vi "Day 11-1.vi"() -> ()   [LabVIEW 2020]
uses:
  <vilib>/regexp/Match Regular Expression.xnode
panel:
  out "Answer":i64
  out "Array":i32[][](array[numeric])
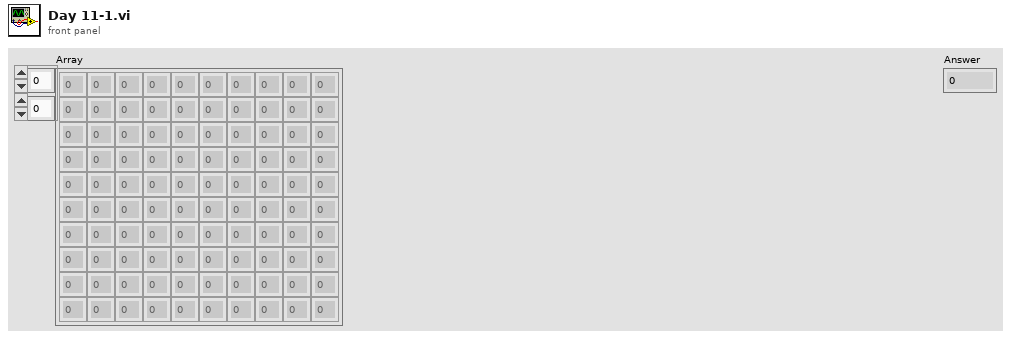
[diagram p1: front panel]
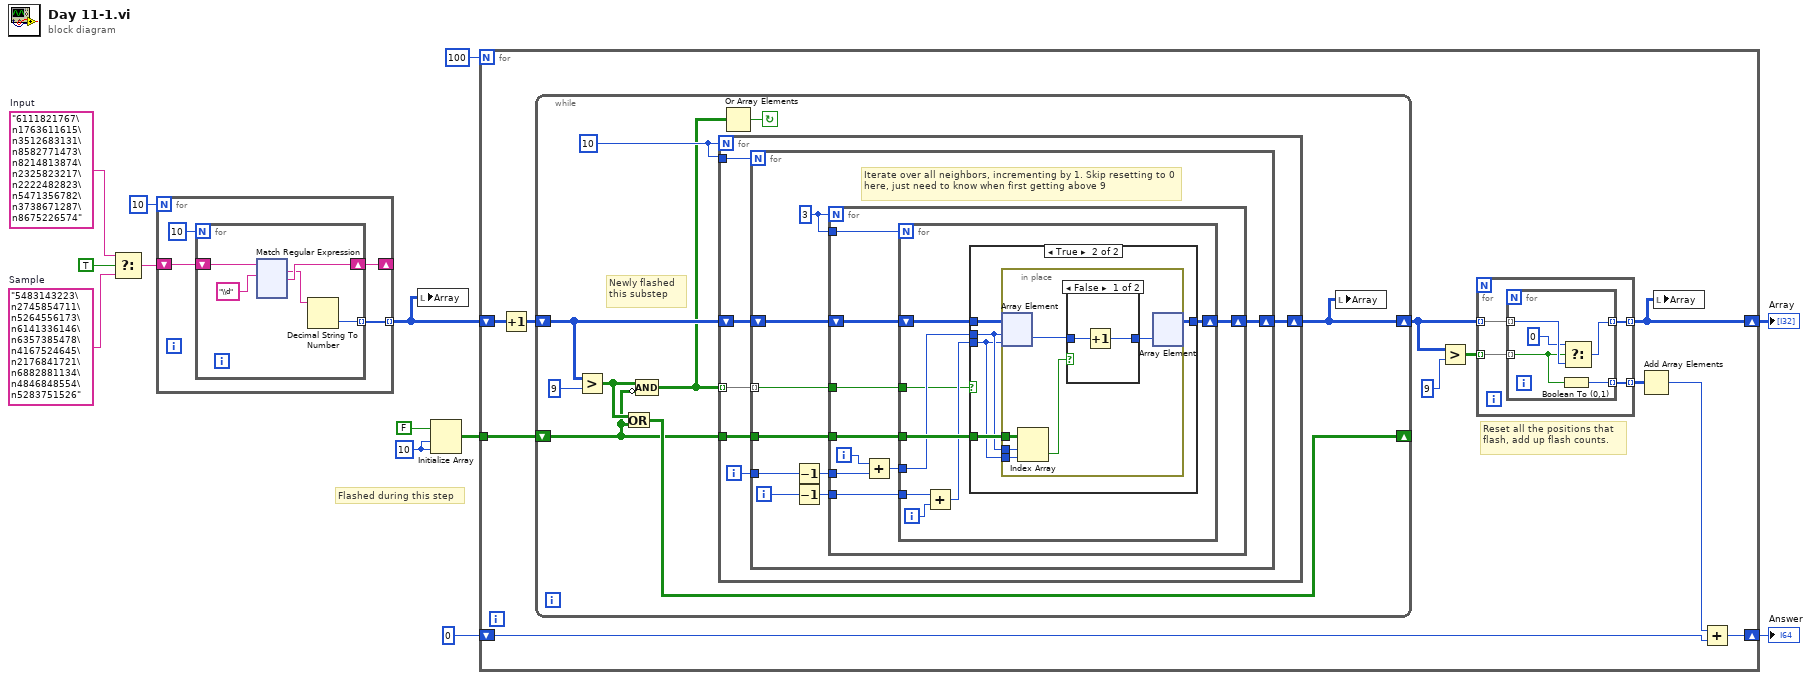
[diagram p0: block diagram]
diagram:
  w4 = 10 ("dimension size")
  w11 = "5483143223\n2745854711\n5264556173\n6141336146\n6357385478\n4167524645\n2176841721\n6882881134\n4846848554\n5283751526"  # Sample
  w12 = "6111821767\n1763611615\n3512683131\n8582771473\n8214813874\n2325823217\n2222482823\n5471356782\n3738671287\n8675226574"  # Input
  # "Flashed during this step"
  n1 = Select(t=w12, s=TRUE, f=w11) -> (s? t:f=w10:string)
  n2 = for {
    N: 10 -> [_]
    shift-right: [w16] -> _
    shift-left: w10 -> [w17]
    tunnel: [w14] -> w1 mode=indexing
    n3 = for {
      N: 10 -> [_]
      shift-right: [w20] -> w16
      shift-left: w17 -> [w22]
      tunnel: [w18] -> w14 mode=indexing
      n4 = xnode "Match Regular Expression"("input string"=w22, "regular expression"="\\d") -> ("whole match"=w19:string, "after match"=w20:string)  [unwired: 4 in, 3 out]
      n5 = Decimal String To Number(string=w19) -> (number=w18:i32)  [unwired: 2 in, 1 out]
    }
  }
  n6 = local write "Array"(w1) -> ()
  n7 = Initialize Array(FALSE, w4, w4) -> (w2:bool[][])
  n8 = for {
    N: 100 -> [_]
    shift-right: [w137] -> w6
    shift-left: w1 -> [w147]
    shift-right: [w140] -> w5
    shift-left: i64 0 -> [w138]
    tunnel: w2 -> [w145]
    # "Reset all the positions that flash, add up flash counts."
    n9 = Increment(x=w147) -> (x+1=w146:i32[][])
    n10 = while {
      shift-right: [w149] -> w143
      shift-left: w146 -> [w154]
      shift-right: [w152] -> _
      shift-left: w145 -> [w150]
      stop <- w155 continue-if-true
      w153 = 10
      # "Newly flashed this substep"
      n11 = Greater?(x=w154, y=9) -> (0:w151:bool[][])
      n12 = Or(x=w151, y=w150) -> (x .or. y?=w152:bool[][])
      n13 = Compound Arithmetic op=AND(w151, invert w150) -> (w148:bool[][])
      n14 = for {
        N: w153 -> [_]
        shift-right: [w160] -> w149
        shift-left: w154 -> [w162]
        tunnel: w148 -> [w161] mode=indexing
        tunnel: w153 -> [w158]
        tunnel: w150 -> [w157]
        i -> [w159]
        n15 = for {
          N: w158 -> [_]
          shift-right: [w171] -> w160
          shift-left: w162 -> [w164]
          tunnel: w159 -> [w170]
          tunnel: w161 -> [w163] mode=indexing
          tunnel: w157 -> [w168]
          i -> [w169]
          w165 = 3
          # "Iterate over all neighbors, incrementing by 1. Skip resetting to 0 here, just need to know when first getting above 9"
          n16 = Decrement(x=w170) -> (x-1=w167:i32)
          n17 = Decrement(x=w169) -> (x-1=w166:i32)
          n18 = for {
            N: w165 -> [_]
            shift-right: [w179] -> w171
            shift-left: w164 -> [w180]
            tunnel: w167 -> [w178]
            tunnel: w166 -> [w177]
            tunnel: w168 -> [w175]
            tunnel: w165 -> [w174]
            tunnel: w163 -> [w172]
            i -> [w173]
            n19 = Add(x=w173, y=w178) -> (x+y=w176:i32)
            n20 = for {
              N: w174 -> [_]
              shift-right: [w186] -> w179
              shift-left: w180 -> [w187]
              tunnel: w176 -> [w184]
              tunnel: w177 -> [w188]
              tunnel: w175 -> [w185]
              tunnel: w172 -> [w181]
              i -> [w182]
              n21 = Add(x=w188, y=w182) -> (x+y=w183:i32)
              n22 = case shown="True" w181 {
                tunnel: w187 -> [w189 w194]
                tunnel: [w189 w193] -> w186
                tunnel: w185 -> [_ w192]
                tunnel: w184 -> [_ w191]
                tunnel: w183 -> [_ w190]
                frame False {
                }
                frame True {
                  n23 = in-place {
                    in-place-border: w192 -> [w198]
                    in-place-border: w191 -> [w197]
                    in-place-border: w190 -> [w196]
                    n24 = in-place-array #1(w194, w191, w190) -> (w200:i32)
                    n25 = Index Array(array=w198, index (row)=w197, index (col)=w196) -> (element=w195:bool)
                    n26 = case shown="False" w195 {
                      tunnel: w200 -> [w202 w203]
                      tunnel: [w201 w203] -> w199
                      frame False {
                        n27 = Increment(x=w202) -> (x+1=w201:i32)
                      }
                      frame True {
                      }
                    }
                    n28 = in-place-array #1(w199) -> (w193:i32[][])  [unwired: 2 out]
                  }
                }
              }
            }
          }
        }
      }
      n29 = Or Array Elements(Boolean array=w148) -> (logical OR=w155:bool)
      n30 = local write "Array"(w149) -> ()
    }
    n31 = Greater?(x=w143, y=9) -> (0:w142:bool[][])
    n32 = for {
      tunnel: w143 -> [w207] mode=indexing
      tunnel: w142 -> [w206] mode=indexing
      tunnel: [w205] -> w141 mode=indexing
      tunnel: [w204] -> w137 mode=indexing
      n33 = for {
        tunnel: w207 -> [w212] mode=indexing
        tunnel: w206 -> [w210] mode=indexing
        tunnel: [w209] -> w205 mode=indexing
        tunnel: [w208] -> w204 mode=indexing
        n34 = Boolean To (0,1)(Boolean=w210) -> (0, 1=w209:i16)
        n35 = Select(t=0, s=w210, f=w212) -> (s? t:f=w208:i32)
      }
    }
    n36 = Add Array Elements(numeric array=w141) -> (sum=w139:i16)
    n37 = local write "Array"(w137) -> ()
    n38 = Add(x=w139, y=w138) -> (x+y=w140:i64)
  }
  "Array" <- w6
  "Answer" <- w5
